vi "Send and Read Next Message_sushu.vi"(0 "Queue In":cluster{"Q":T1, "Name":string}, 1 "Elements at Back":string, 3 "timeout (1 ms)":i32=1, 4 "message value input":string, 5 "error in":errorcluster, 6 "receiver process (\"\" - local)":string, 8 "Elements in Front":string) -> (7 "acknowledge":bool, 10 "Previous State + Arguments":string, 11 "timed out?":bool, 12 "exit process?":bool, 13 "message":T2, 14 "Queue Out":cluster{"Q":T1, "Name":string}, 15 "Arguments":string, 16 "message value":string, 17 "Current State":string, 19 "error out":errorcluster)   [LabVIEW 2021]
doc: "基于AMC二次封装的读取队列元素的模块。\n20140304\nReturns the next message from the message queue passed in. If the returned message matches any of the message names listed in \"termination list\" the \"exit process?\" indicator will return True."
uses:
  <vilib>/NI/AMC/AMC.lvlib
  <vilib>/NI/AMC/Message.ctl
  <vilib>/NI/AMC/Message Queue.ctl
  <vilib>/NI/Tools/Keyed Array/KeyedArray.ctl
  <vilib>/NI/Tools/Keyed Array/Tools_KeyedArray.lvlib
panel:
  in  "ignore error on termination message (F)":bool
  in  "termination list ([Exit])":string[](array[string])=["Exit"]
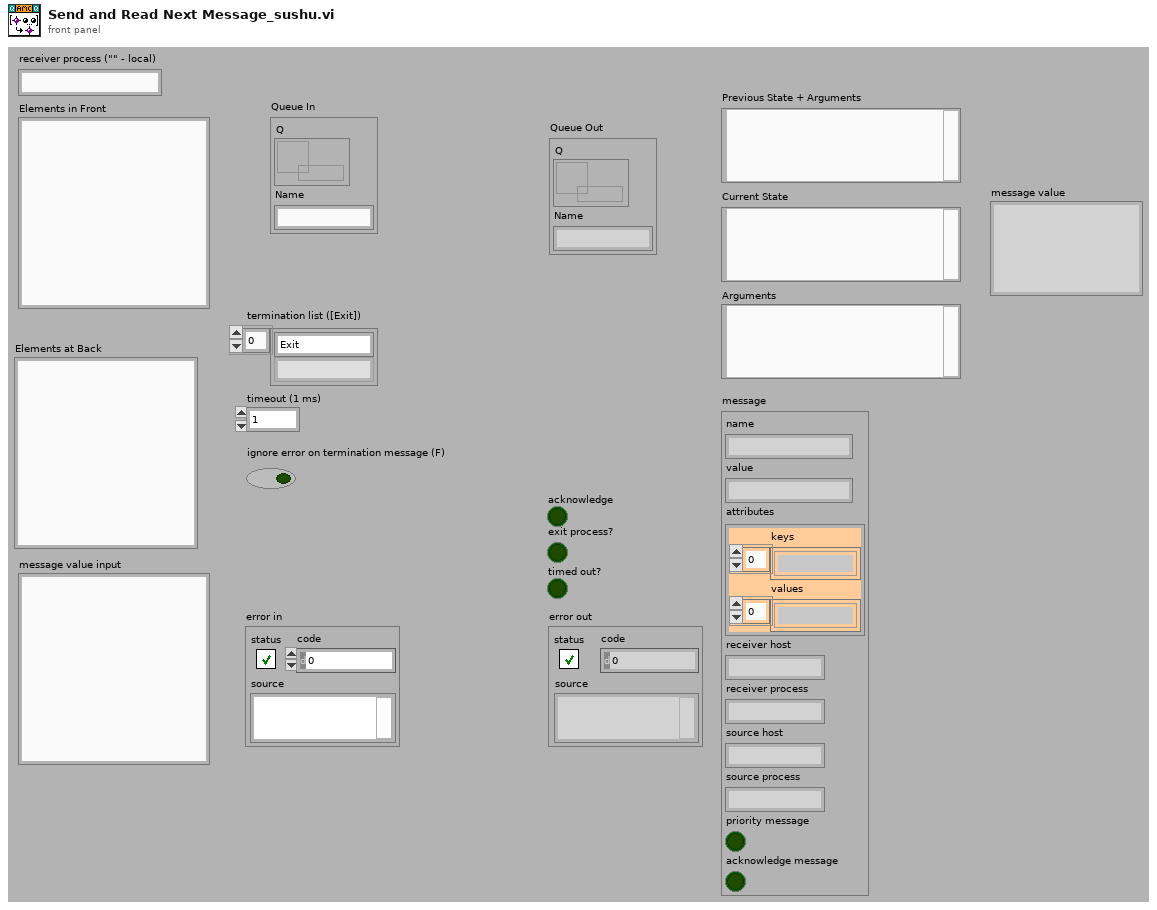
[diagram p1: front panel]
types:
  T1 = typedef "AMC.lvlib/Message Queue.ctl" = refnum<queue>
  T2 = typedef "AMC.lvlib/Message.ctl" = cluster{"name":string, "value":string, "attributes":T3, "receiver host":string, "receiver process":string, "source host":string, "source process":string, "priority message":bool, "acknowledge message":bool}
  T3 = typedef "Tools_KeyedArray.lvlib/KeyedArray.ctl" = cluster{"keys":string[], "values":string[]}
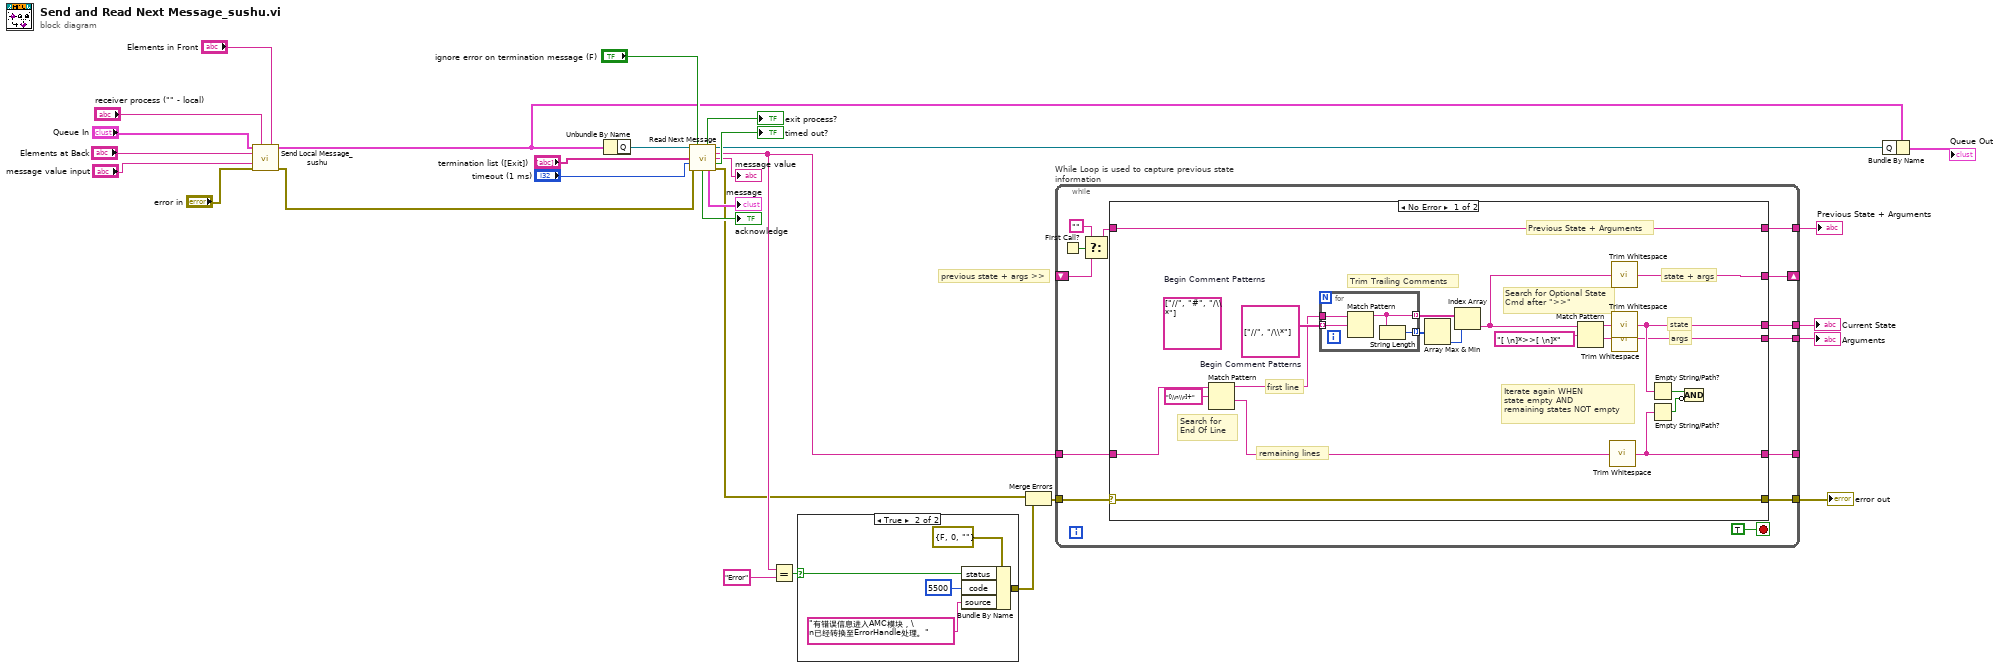
[diagram p0: block diagram]
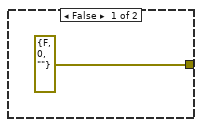
[diagram p2: hidden frame]
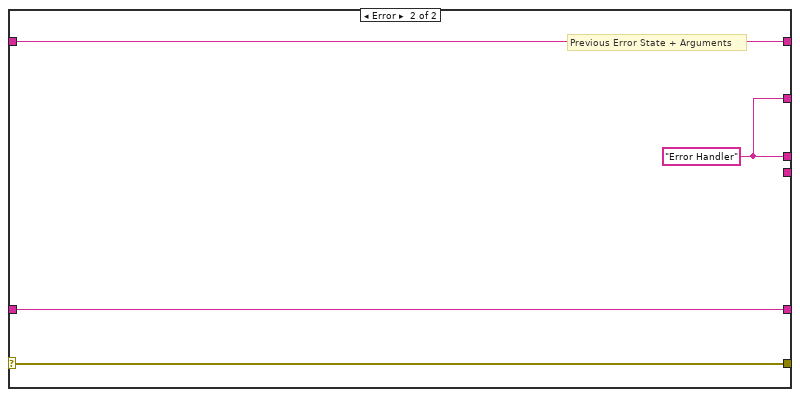
[diagram p3: hidden frame]
diagram:
  # "previous state + args >>"
  n1 = call <userlib>:"Send Local Message_sushu.vi"("Queue In"="Queue In", "receiver process (\"\" - local)"="receiver process (\"\" - local)", "Elements in Front"="Elements in Front", "Elements at Back"="Elements at Back", "message value"="message value input", "error in"="error in") -> ("Queue Out"=w5:cluster{"Q":T1, "Name":string}, "error out"=w4:errorcluster)  [unwired: 7 in, 1 out]
  n2 = Unbundle By Name(w5) -> ("Q"=w21:T1)
  n3 = call <vilib>:"Read Next Message.vi"("message queue in"=w21, "ignore error on termination message (F)"="ignore error on termination message (F)", "termination list ([Exit])"="termination list ([Exit])", "timeout (1 ms)"="timeout (1 ms)", "error in"=w4) -> ("exit process?"=→"exit process?":bool, "message queue out"=w20:T1, "message name"=w14:string, "message value"=→"message value":string, "timed out?"=→"timed out?":bool, "acknowledge"=→"acknowledge":bool, "message"=→"message":T2, "error out"=w11:errorcluster)  [unwired: 3 in]
  n4 = Equal?(x=w14, y="Error") -> (x = y?=w10:bool)
  n5 = case shown="True" w10 {
    selector: w10 -> [_ w32]
    tunnel: [errorcluster {"status"=FALSE, "code"=0, "source"=""} ("error constant") w31] -> w9
    frame False {
    }
    frame True {
      n6 = Bundle By Name(cluster=errorcluster {"status"=FALSE, "code"=0, "source"=""} ("error constant"), "status"=w32, "code"=5500, "source"="有错误信息进入AMC模块，\n已经转换至ErrorHandle处理。") -> (w31:errorcluster)
    }
  }
  n7 = Merge Errors(w11, w9) -> (w12:errorcluster)
  n8 = while "While Loop is used to capture previous state information" {
    tunnel: [w48] -> _
    tunnel: w14 -> [w47]
    tunnel: w12 -> [w46]
    tunnel: [w45] -> w18
    tunnel: [w44] -> w17
    shift-right: [w42] -> _
    shift-left: _ -> [w40]
    tunnel: [w37] -> w16
    tunnel: [w36] -> w15
    stop <- TRUE stop-if-true
    n9 = First Call?() -> (First Call?: T/F=w41:bool)
    n10 = Select(t="", s=w41, f=w40) -> (s? t:f=w39:string)
    n11 = case shown="No Error" w46 {
      selector: w46 -> [w62 w73]
      tunnel: [w65 w76] -> w48
      tunnel: [w68 w74] -> w45
      tunnel: [w67 _] -> w44
      tunnel: w47 -> [w66 w76]
      tunnel: [w64 w74] -> w42
      tunnel: w39 -> [w63 w75]
      tunnel: [w63 w75] -> w37
      tunnel: [w62 w73] -> w36
      frame No Error {
        (unwired) string[] ["//", "#", "/\\*"]  # Begin Comment Patterns
        w60 = string[] ["//", "/\\*"]  # Begin Comment Patterns
        # "state + args"
        # "remaining lines"
        # "first line"
        # "Search for End Of Line"
        # "Iterate again WHEN\nstate empty AND\nremaining states NOT empty"
        # "args"
        # "state"
        # "Search for Optional State Cmd after \">>\""
        # "Trim Trailing Comments"
        # "Previous State + Arguments"
        n12 = Match Pattern(string=w66, regular expression="[\\n\\r]+") -> (before substring=w50:string, after substring=w61:string)  [unwired: 1 in, 2 out]
        n13 = for {
          tunnel: w50 -> [w72]
          tunnel: [w70] -> w57 mode=indexing
          tunnel: w60 -> [w71] mode=indexing
          tunnel: [w69] -> w59 mode=indexing
          n14 = Match Pattern(string=w72, regular expression=w71) -> (before substring=w70:string)  [unwired: 1 in, 3 out]
          n15 = String Length(string=w70) -> (length=w69:i32)
        }
        n16 = Array Max & Min(array=w59) -> (min index (indices)=w58:i32)  [unwired: 3 out]
        n17 = Index Array(array=w57, index=w58) -> (element=w49:string)
        n18 = Match Pattern(string=w49, regular expression="[ \n]*>>[ \n]*") -> (before substring=w55:string, after substring=w54:string)  [unwired: 1 in, 2 out]
        n19 = call <vilib>:"Trim Whitespace.vi"("string"=w61) -> ("trimmed string"=w65:string)  [unwired: 1 in]
        n20 = call <vilib>:"Trim Whitespace.vi"("string"=w49) -> ("trimmed string"=w64:string)  [unwired: 1 in]
        n21 = call <vilib>:"Trim Whitespace.vi"("string"=w55) -> ("trimmed string"=w68:string)  [unwired: 1 in]
        n22 = call <vilib>:"Trim Whitespace.vi"("string"=w54) -> ("trimmed string"=w67:string)  [unwired: 1 in]
        n23 = Empty String/Path?(string/path=w68) -> (empty?=w53:bool)
        n24 = Empty String/Path?(string/path=w65) -> (empty?=w52:bool)
        n25 = Compound Arithmetic op=AND(w53, invert w52) -> ()  [unwired: 1 out]
      }
      frame Error {
        w74 = "Error Handler"
        # "Previous Error State + Arguments"
      }
    }
  }
  "error out" <- w15
  "Arguments" <- w17
  "Current State" <- w18
  "Previous State + Arguments" <- w16
  n26 = Bundle By Name(cluster=w5, "Q"=w20) -> (→"Queue Out":cluster{"Q":T1, "Name":string})
